vi "I2C Tap Bridge.vi"(0 "input channel i2c io":T2, 1 "reset":bool, 5 "output channel i2c io":T2, 12 "enable i2c tap bridge":bool) -> (4 "i2c monitor":T1 {"monitor word" format="%.0x"})   [LabVIEW 2020, in "GettingStarted_Common_148X_FPGA.lvlib"]
uses:
  GettingStarted_Common_148X_FPGA.lvlib
  Types/I2C IO.ctl
  <instrlib>/FlexRIO/API/FPGA/v1/IO/NI148x/i2c monitor.ctl
  <instrlib>/FlexRIO/API/FPGA/v1/IO/NI148x/Single I2C In.ctl
  <vilib>/rvi/eio/common/nirviEmuTemplateMethod_errors.vi
  <vilib>/eio/EIONode/EIONode.xnode
  <instrlib>/FlexRIO/API/FPGA/v1/IO/NI148x/FlexRIO 148x FPGA v1.lvlib
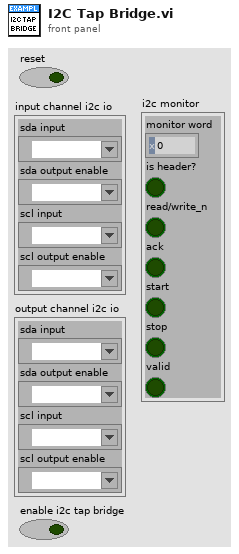
[diagram p1: front panel]
types:
  T1 = typedef "FlexRIO 148x FPGA v1.lvlib/i2c monitor.ctl" = cluster{"monitor word":u8, "is header?":bool, "read/write_n":bool, "ack":bool, "start":bool, "stop":bool, "valid":bool}
  T2 = typedef "GettingStarted_Common_148X_FPGA.lvlib/I2C IO.ctl" = cluster{"sda input":refnum<k21>, "sda output enable":refnum<k21>, "scl input":refnum<k21>, "scl output enable":refnum<k21>}
  T3 = typedef "FlexRIO 148x FPGA v1.lvlib/Single I2C In.ctl" = cluster{"SCL_I":bool, "SDA_I":bool}
  T4 = typedef "FlexRIO 148x FPGA v1.lvlib/Single I2C Out.ctl" = cluster{"SCL_OE":bool, "SDA_OE":bool}
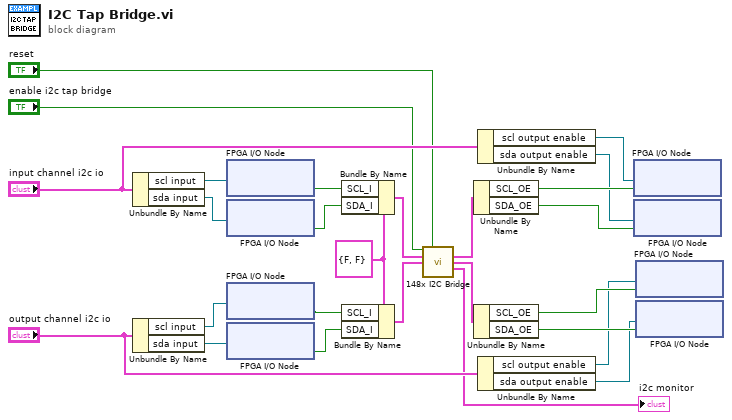
[diagram p0: block diagram]
diagram:
  w17 = T3 {"SCL_I"=FALSE, "SDA_I"=FALSE} ("i2c 0 in")
  n1 = Unbundle By Name("input channel i2c io") -> ("scl input"=w7:refnum<k21>, "sda input"=w5:refnum<k21>)
  n2 = Unbundle By Name("output channel i2c io") -> ("scl input"=w13:refnum<k21>, "sda input"=w14:refnum<k21>)
  n3 = xnode "FPGA I/O Node"("FPGA I/O In"=w7) -> ("I/O Item"=w3:bool)  [unwired: 1 out]
  n4 = xnode "FPGA I/O Node"("FPGA I/O In"=w5) -> ("I/O Item"=w4:bool)  [unwired: 1 out]
  n5 = xnode "FPGA I/O Node"("FPGA I/O In"=w13) -> ("I/O Item"=w15:bool)  [unwired: 1 out]
  n6 = xnode "FPGA I/O Node"("FPGA I/O In"=w14) -> ("I/O Item"=w16:bool)  [unwired: 1 out]
  n7 = Bundle By Name(cluster=w17, "SCL_I"=w3, "SDA_I"=w4) -> (w6:T3)
  n8 = Bundle By Name(cluster=w17, "SCL_I"=w15, "SDA_I"=w16) -> (w23:T3)
  n9 = call <instrlib>:"148x I2C Bridge.vi"("enable tap bridge"="enable i2c tap bridge", "reset"="reset", "i2c 0 in"=w6, "i2c 1 in"=w23) -> ("i2c 0 out"=w8:T4, "i2c 1 out"=w24:T4, "i2c monitor"=→"i2c monitor":T1)  [unwired: 9 in]
  n10 = Unbundle By Name(w8) -> ("SCL_OE"=w11:bool, "SDA_OE"=w12:bool)
  n11 = Unbundle By Name(w24) -> ("SCL_OE"=w21:bool, "SDA_OE"=w22:bool)
  n12 = Unbundle By Name("input channel i2c io") -> ("scl output enable"=w9:refnum<k21>, "sda output enable"=w10:refnum<k21>)
  n13 = Unbundle By Name("output channel i2c io") -> ("scl output enable"=w18:refnum<k21>, "sda output enable"=w19:refnum<k21>)
  n14 = xnode "FPGA I/O Node"("I/O Item"=w11, "FPGA I/O In"=w9) -> ()  [unwired: 1 out]
  n15 = xnode "FPGA I/O Node"("I/O Item"=w12, "FPGA I/O In"=w10) -> ()  [unwired: 1 out]
  n16 = xnode "FPGA I/O Node"("I/O Item"=w21, "FPGA I/O In"=w18) -> ()  [unwired: 1 out]
  n17 = xnode "FPGA I/O Node"("I/O Item"=w22, "FPGA I/O In"=w19) -> ()  [unwired: 1 out]
